vi "batch callbyref wait on all.vi"() -> ()   [LabVIEW 2013]
uses:
  result/result.lvclass
  result/result.lvclass/result.ctl
  result/get data.vi
  result/get error.vi
  result/get generating action.vi
  result/get owning task.vi
  result/get subresults.vi
  standard action/call by reference action/invoke reentrant method in parallel.vi
  dispatcher/thread pool.lvclass
  standard reporters/event reporter/event reporter.lvclass
  standard action/call by reference action/call by reference action.lvclass
panel:
  out "owning task":string
  out "generating action":string
  out "error":errorcluster
  out "data":variant
  out "actions":string[](array[string])
  out "Array 2":errorcluster[](array[cluster])
  out "Array":variant[](array[variant])
  out "Time":u32
  out "result":refnum<class "result.lvclass">
  out "error out":errorcluster
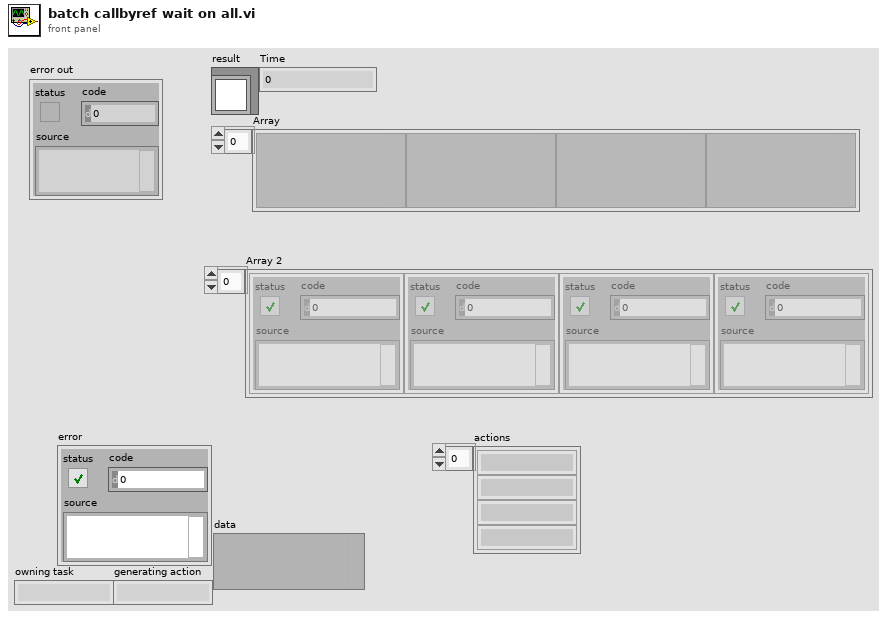
[diagram p1: front panel]
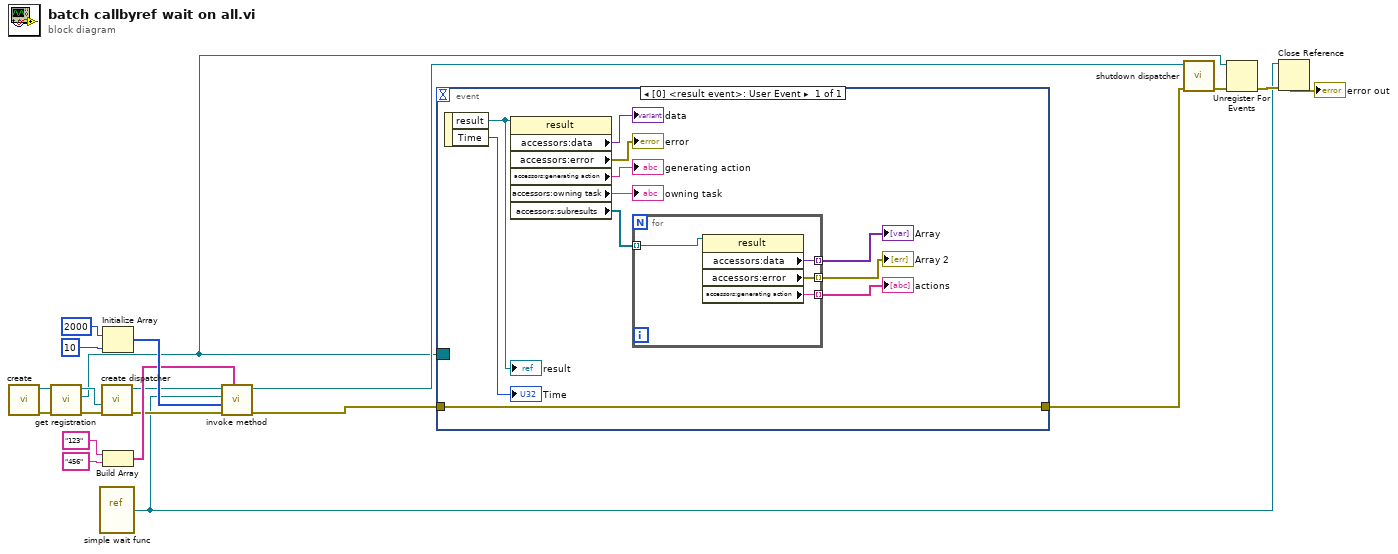
[diagram p0: block diagram]
diagram:
  n1 = call "create.vi"() -> ("error out"=w19:errorcluster, "event reporter out"=w20:refnum<class "event reporter.lvclass">)  [unwired: 10 in]
  n2 = call "get registration.vi"("error in"=w19, "event reporter in"=w20) -> ("error out"=w17:errorcluster, "result registration"=w1:refnum<event-registration>, "event reporter out"=w18:refnum<class "event reporter.lvclass">)  [unwired: 7 in]
  n3 = vi-ref "simple wait func.vi"() -> (w2:refnum<vi>)
  n4 = call "create dispatcher.vi"("error in"=w17, "default reporter"=w18) -> ("error out"=w7:errorcluster, "dispatcher"=w4:refnum<data-value>)  [unwired: 8 in]
  n5 = Initialize Array(2000, 10 ("dimension size")) -> (w11:i32[])
  n6 = Build Array("123" ("ID"), "456" ("element")) -> (w9:string[])
  n7 = call-poly "invoke method.vi"("IDs"=w9, "error in"=w7, "parameters"=w11, "VI in"=w2, "dispatcher"=w4) -> ("error out"=w6:errorcluster, "dispatcher out"=w5:refnum<data-value>)  [unwired: 5 in]
  n8 = event shown="[0] <result event>: User Event" {
    selector: w1 -> [_]
    dyn-events: _ -> [_]
    timeout: _ -> [_]
    tunnel: [w30] -> w14
    tunnel: w6 -> [w30]
    event User Event {
      n9 = event-data() -> ("result"=w29:refnum<class "result.lvclass">, "Time"=→"Time":u32)  [unwired: 1 in]
      "result" <- w29
      n10 = property class="result"(reference=w29) -> ("accessors:data"=→"data":variant, "accessors:error"=→"error":errorcluster, "accessors:generating action"=→"generating action":string, "accessors:owning task"=→"owning task":string, "accessors:subresults"=w28:refnum<class "result.lvclass">[])  [unwired: 1 in, 2 out]
      n11 = for {
        tunnel: w28 -> [w35] mode=indexing
        tunnel: [w34] -> w27 mode=indexing
        tunnel: [w33] -> w26 mode=indexing
        tunnel: [w32] -> w25 mode=indexing
        n12 = property class="result"(reference=w35) -> ("accessors:data"=w34:variant, "accessors:error"=w33:errorcluster, "accessors:generating action"=w32:string)  [unwired: 1 in, 2 out]
      }
      "Array" <- w27
      "Array 2" <- w26
      "actions" <- w25
    }
  }
  n13 = call "shutdown dispatcher.vi"("error in"=w14, "dispatcher"=w5) -> ("error out"=w16:errorcluster)  [unwired: 9 in]
  n14 = Unregister For Events(event registration refnum=w1, error in=w16) -> (error out=w15:errorcluster)
  n15 = Close Reference(reference=w2, error in (no error)=w15) -> (error out=→"error out":errorcluster)
